vi "Panel Timeout Helper.vi"(7 "Visible mS":i32, 8 "Update?":bool, 9 "Visible?":bool) -> (3 "Timeout":i32)   [LabVIEW 2018, in "OOPanel.lvlib" / "Panel.lvclass"]
uses:
  Panel.lvclass
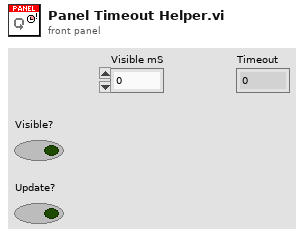
[diagram p1: front panel]
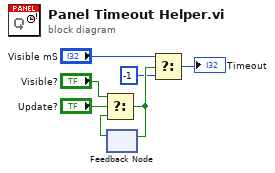
[diagram p0: block diagram]
diagram:
  n1 = feedback #1() -> (w5:bool)  [unwired: 1 in]
  n2 = Select(t="Visible?", s="Update?", f=w5) -> (s? t:f=w4:bool)
  n3 = feedback-in #1(w4) -> ()
  n4 = Select(t="Visible mS", s=w4, f=-1) -> (s? t:f=→"Timeout":i32)
